vi "OpenPanels.vi"(6 "Spike":string, 7 "Single?":bool, 8 "File Name":string, 9 "Backpack":string, 10 "Code":string, 11 "VI in":refnum<vi>) -> ()   [LabVIEW 2016]
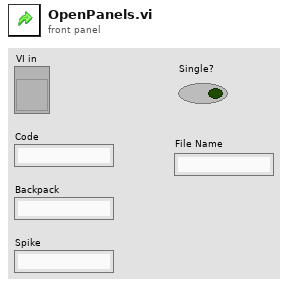
[diagram p1: front panel]
types:
  T1 = enum32{"Invalid", "Standard", "Closed", "Hidden", "Minimized", "Maximized"}
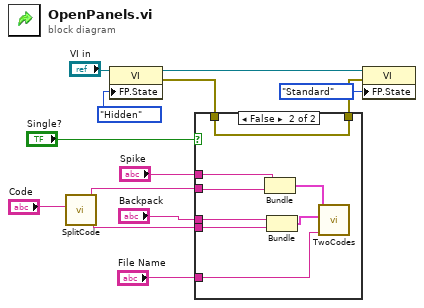
[diagram p0: block diagram]
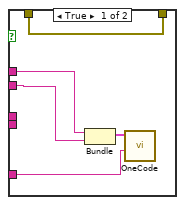
[diagram p2: hidden frame]
diagram:
  n1 = call "SplitCode.vi"("Code"="Code") -> ("BP Code"=w1:string, "Spike Code"=w5:string)  [unwired: 9 in]
  n2 = property class="VI"(reference="VI in", "FP.State"=T1."Hidden" ("Front Panel Window:State")) -> (reference out=w10:refnum<vi>, error out=w8:errorcluster)  [unwired: 1 in]
  n3 = case shown="False" "Single?" {
    tunnel: [w18 w26] -> w9
    tunnel: w8 -> [w18 w26]
    tunnel: "Spike" -> [w17 w25]
    tunnel: "Backpack" -> [_ w23]
    tunnel: w5 -> [w15 w22]
    tunnel: "File Name" -> [w16 w21]
    tunnel: w1 -> [_ w20]
    frame True {
      n4 = Bundle("Spike"=w17, "Spike Code"=w15) -> (w14:cluster{"Spike":string, "Spike Code":string})  [unwired: 1 in]
      n5 = call "OneCode.vi"("VI Name"=w16, "Default"=w14) -> ()  [unwired: 10 in]
    }
    frame False {
      n6 = Bundle("Spike"=w25, "Spike Code"=w22) -> (w24:cluster{"Spike":string, "Spike Code":string})  [unwired: 1 in]
      n7 = Bundle("Backpack"=w23, "BP Code"=w20) -> (w19:cluster{"Backpack":string, "BP Code":string})  [unwired: 1 in]
      n8 = call "TwoCodes.vi"("VI Name"=w21, "Backpack"=w19, "Spike"=w24) -> ()  [unwired: 9 in]
    }
  }
  n9 = property class="VI"(reference=w10, error in=w9, "FP.State"=T1."Standard" ("Front Panel Window:State")) -> ()  [unwired: 2 out]
